vi "CCExcelToDcmGenerateUIDs.vi"(11 "String in":string) -> (3 "String out":string)   [LabVIEW 2013, in "main.lvlib" / "ClearCanvasLibrary.lvlib"]
uses:
  ClearCanvasLibrary.lvlib
  C:/Users/Simon/SkyDrive/LabView/2013/DM2020/DICOM/ClearCanvasNewBuild/ClearCanvas.Dicom.dll
  ClearCanvasNewBuild/ClearCanvas.Dicom.dll
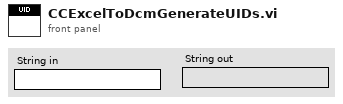
[diagram p1: front panel]
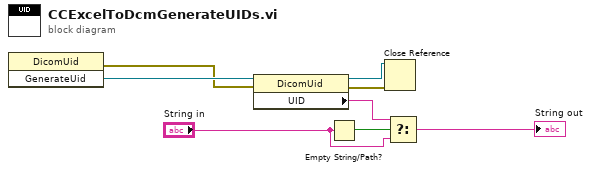
[diagram p0: block diagram]
diagram:
  n1 = invoke class="DicomUid" method="GenerateUid"() -> (error out=w3:errorcluster, "GenerateUid"=w4:refnum<k24>)  [unwired: 3 in, 1 out]
  n2 = property class="DicomUid"(reference=w4, error in=w3) -> (reference out=w6:refnum<k24>, error out=w7:errorcluster, "UID"=w8:string)
  n3 = Empty String/Path?(string/path="String in") -> (empty?=w5:bool)
  n4 = Close Reference(reference=w6, error in (no error)=w7) -> ()  [unwired: 1 out]
  n5 = Select(t=w8, s=w5, f="String in") -> (s? t:f=→"String out":string)
